vi "resetOutput.vi"(8 "error in (no error)":errorcluster, 11 "k3390_AWG in":refnum<class "k3390_AWG.lvclass">) -> (0 "error out":errorcluster, 3 "k3390_AWG out":refnum<class "k3390_AWG.lvclass">)   [LabVIEW 2009, in "Hardware.lvlib" / "Channels.lvlib" / "k3390_AWG.lvclass"]
uses:
  k3390_AWG.lvclass
  Generic/DDSOutput.lvclass
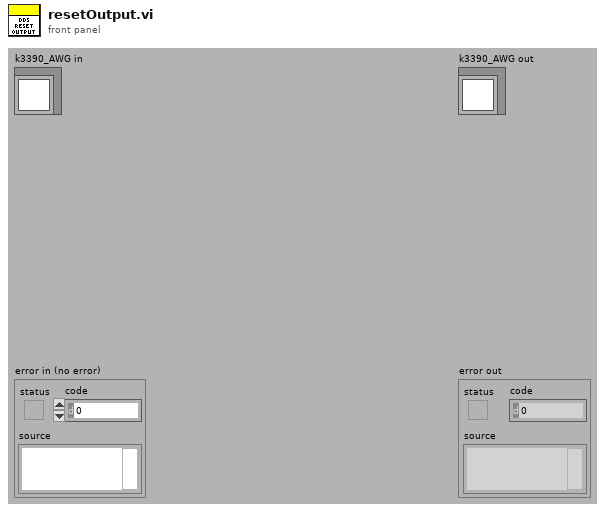
[diagram p1: front panel]
types:
  T1 = cluster{"Frequency(MHz)":dbl, "Amplitude":dbl, "Phase":dbl, "OutputForm":enum16{"Sine", "Square", "Triangle", "Arbitrary"}}[]
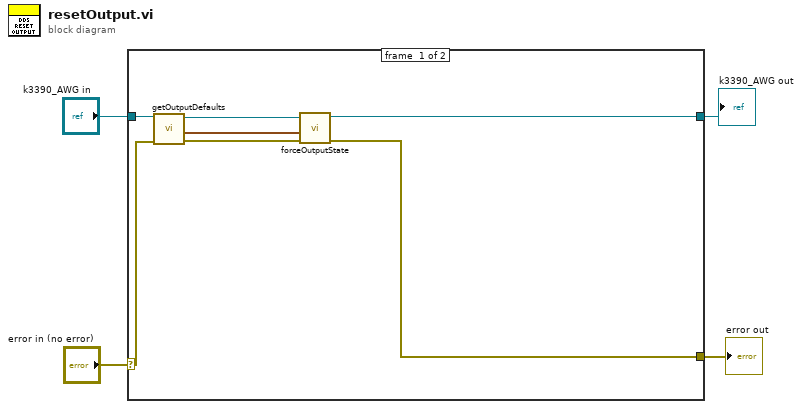
[diagram p0: block diagram]
diagram:
  n1 = case shown="No Error" "error in (no error)" {
    selector: "error in (no error)" -> [w10 w12]
    tunnel: "k3390_AWG in" -> [w11 w13]
    tunnel: [w6 w13] -> w2
    tunnel: [w5 w12] -> w1
    frame #0 {
      n2 = call "getOutputDefaults.vi"("error in (no error)"=w10, "DDSOutput in"=w11) -> ("error out"=w7:errorcluster, "Defaults"=w8:T1, "DDSOutput out"=w9:refnum<class "k3390_AWG.lvclass">)  [unwired: 6 in, 1 out]
      n3 = call-dynamic "forceOutputState.vi"("error in (no error)"=w7, "data"=w8, "k3390_AWG in"=w9) -> ("error out"=w5:errorcluster, "k3390_AWG out"=w6:refnum<class "k3390_AWG.lvclass">)  [unwired: 7 in]
    }
    frame #1 {
    }
  }
  "error out" <- w1
  "k3390_AWG out" <- w2
